vi "Read from File.vi"(7 "Section Name":string, 8 "error in (no error)":errorcluster, 10 "INI Ref":T1, 11 "Step in":refnum<class "Step.lvclass">) -> (0 "error out":errorcluster, 2 "INI Ref out":T1, 3 "Step out":refnum<class "Step.lvclass">)   [LabVIEW 2020, in "MacroAssert.lvlib" / "Step.lvclass"]
doc: "Reads associated parameters from the file identified by <B>INI Ref</B>."
uses:
  Step.lvclass
  <vilib>/Utility/config.llb/Config Data RefNum.ctl
  CTLs/Step Type v1.ctl
  <vilib>/Utility/error.llb/Error Cluster From Error Code.vi
  <vilib>/Utility/config.llb/Read Key (String).vi
  <vilib>/Utility/config.llb/Read Key (I32).vi
  <vilib>/Utility/config.llb/Read Key (Boolean).vi
  SubVIs/Custom Errors/Custom Errors.lvlib
  <vilib>/Utility/config.llb/NI_LVConfig.lvlib
  MacroAssert.lvlib
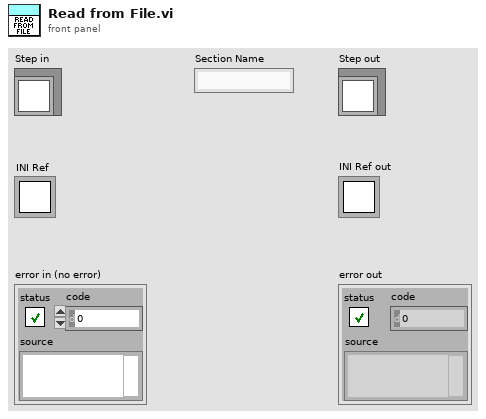
[diagram p1: front panel]
types:
  T1 = typedef "NI_LVConfig.lvlib/Config Data RefNum.ctl" = refnum<k1>
  T2 = typedef "MacroAssert.lvlib/Step Type v1.ctl" = enum16{"Mouse Action", "Keyboard Action", "Window Action", "Timing Action", "Boolean Assertion", "Numeric Assertion", "String Assertion", "Image Assertion"}
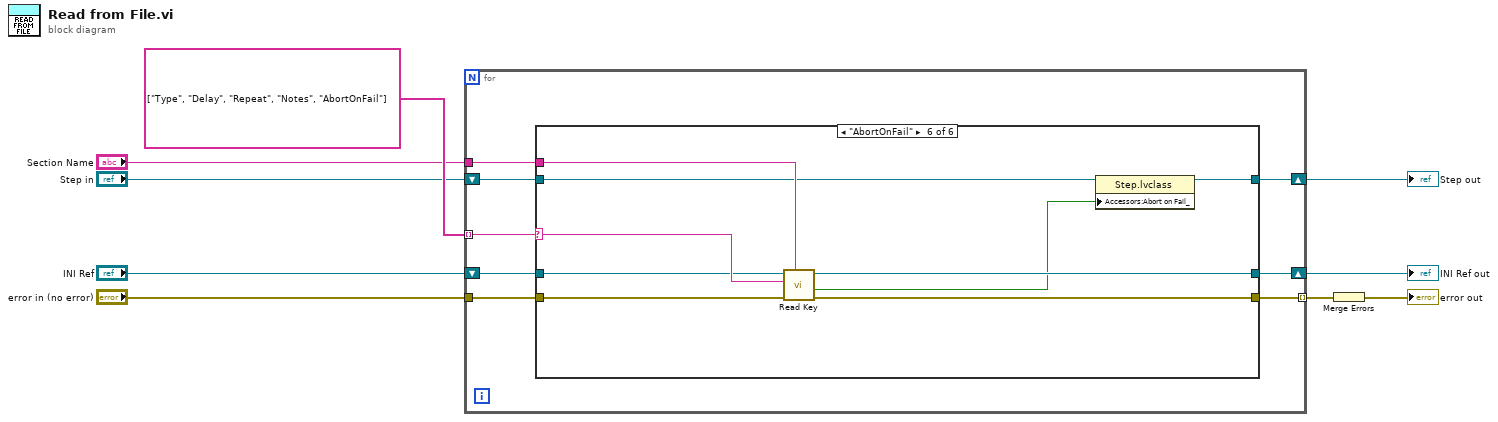
[diagram p0: block diagram]
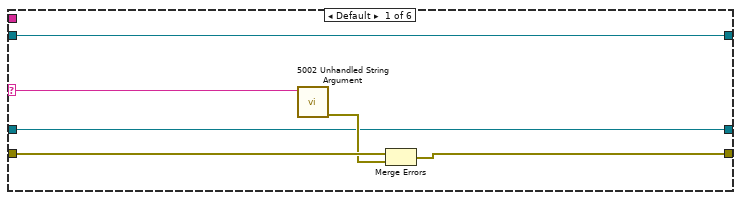
[diagram p2: hidden frame]
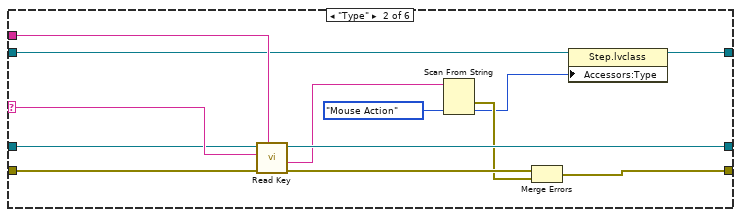
[diagram p3: hidden frame]
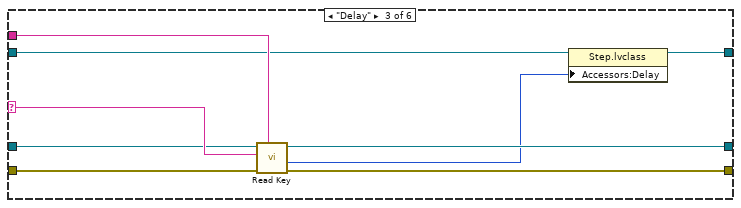
[diagram p4: hidden frame]
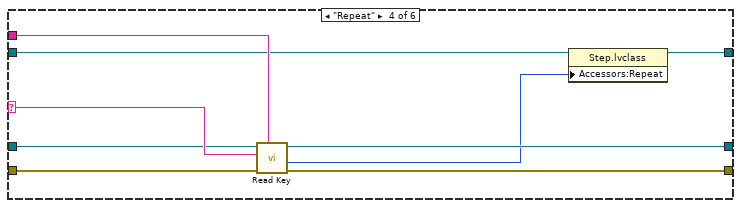
[diagram p5: hidden frame]
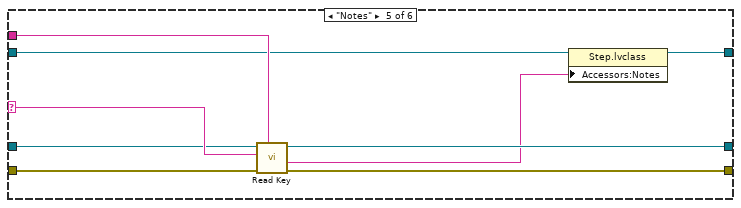
[diagram p6: hidden frame]
diagram:
  n1 = for {
    tunnel: string[] ["Type", "Delay", "Repeat", "Notes", "AbortOnFail"] -> [w17] mode=indexing
    tunnel: "error in (no error)" -> [w16]
    tunnel: "Section Name" -> [w15]
    shift-right: [w13] -> w2
    shift-left: "Step in" -> [w14]
    tunnel: [w12] -> w8 mode=indexing
    shift-right: [w10] -> w3
    shift-left: "INI Ref" -> [w11]
    n2 = case shown="\"AbortOnFail\"" w17 {
      selector: w17 -> [w20 w31 w40 w49 w58 w67]
      tunnel: w16 -> [w22 w36 w45 w54 w63 w72]
      tunnel: w15 -> [_ w35 w44 w53 w62 w71]
      tunnel: w14 -> [w23 w34 w43 w52 w61 w70]
      tunnel: [w23 w33 w42 w51 w60 w69] -> w13
      tunnel: [w19 w27 w41 w50 w59 w68] -> w12
      tunnel: w11 -> [w18 w30 w39 w48 w57 w66]
      tunnel: [w18 w29 w38 w47 w56 w65] -> w10
      frame Default {
        n3 = call "5002 Unhandled String Argument.vi"("Argument"=w20) -> ("error out"=w21:errorcluster)  [unwired: 10 in]
        n4 = Merge Errors(w22, w21) -> (w19:errorcluster)
      }
      frame "Type" {
        n5 = call-poly <vilib>:"Read Key.vi"("section"=w35, "error in (no error)"=w36, "key"=w31, "refnum"=w30) -> ("error out"=w32:errorcluster, "value"=w28:string, "refnum out"=w29:T1)  [unwired: 4 in, 1 out]
        n6 = Scan From String(input string=w28, default 1=Step_Type_v1."Mouse Action" ("Step Type")) -> (error out=w26:errorcluster, output 1=w25:T2)  [unwired: 3 in, 2 out]
        n7 = Merge Errors(w32, w26) -> (w27:errorcluster)
        n8 = property class="Step.lvclass"(reference=w34, "Accessors:Type"=w25) -> (reference out=w33:refnum<class "Step.lvclass">)  [unwired: 1 in, 1 out]
      }
      frame "Delay" {
        n9 = call-poly <vilib>:"Read Key.vi"("section"=w44, "error in (no error)"=w45, "key"=w40, "refnum"=w39) -> ("error out"=w41:errorcluster, "value"=w37:i32, "refnum out"=w38:T1)  [unwired: 4 in, 1 out]
        n10 = property class="Step.lvclass"(reference=w43, "Accessors:Delay"=w37) -> (reference out=w42:refnum<class "Step.lvclass">)  [unwired: 1 in, 1 out]
      }
      frame "Repeat" {
        n11 = call-poly <vilib>:"Read Key.vi"("section"=w53, "error in (no error)"=w54, "key"=w49, "refnum"=w48) -> ("error out"=w50:errorcluster, "value"=w46:i32, "refnum out"=w47:T1)  [unwired: 4 in, 1 out]
        n12 = property class="Step.lvclass"(reference=w52, "Accessors:Repeat"=w46) -> (reference out=w51:refnum<class "Step.lvclass">)  [unwired: 1 in, 1 out]
      }
      frame "Notes" {
        n13 = call-poly <vilib>:"Read Key.vi"("section"=w62, "error in (no error)"=w63, "key"=w58, "refnum"=w57) -> ("error out"=w59:errorcluster, "value"=w55:string, "refnum out"=w56:T1)  [unwired: 4 in, 1 out]
        n14 = property class="Step.lvclass"(reference=w61, "Accessors:Notes"=w55) -> (reference out=w60:refnum<class "Step.lvclass">)  [unwired: 1 in, 1 out]
      }
      frame "AbortOnFail" {
        n15 = call-poly <vilib>:"Read Key.vi"("section"=w71, "error in (no error)"=w72, "key"=w67, "refnum"=w66) -> ("error out"=w68:errorcluster, "value"=w64:bool, "refnum out"=w65:T1)  [unwired: 4 in, 1 out]
        n16 = property class="Step.lvclass"(reference=w70, "Accessors:Abort on Fail_"=w64) -> (reference out=w69:refnum<class "Step.lvclass">)  [unwired: 1 in, 1 out]
      }
    }
  }
  "Step out" <- w2
  "INI Ref out" <- w3
  n17 = Merge Errors(w8) -> (→"error out":errorcluster)
